vi "GUI Update Value.vi"(6 "Time":dbl, 8 "error in (no error)":errorcluster, 11 "GUI Element in":refnum<class "GUI Element.lvclass">) -> (0 "error out":errorcluster, 2 "Update":bool, 3 "GUI Element out":refnum<class "GUI Element.lvclass">, 5 "Value":variant, 7 "Control Index":i32)   [LabVIEW 2020, in "VolatusGUI.lvlib" / "GUI Element.lvclass"]
uses:
  GUI Element.lvclass
  GUI Element.lvclass/GUI Element.ctl
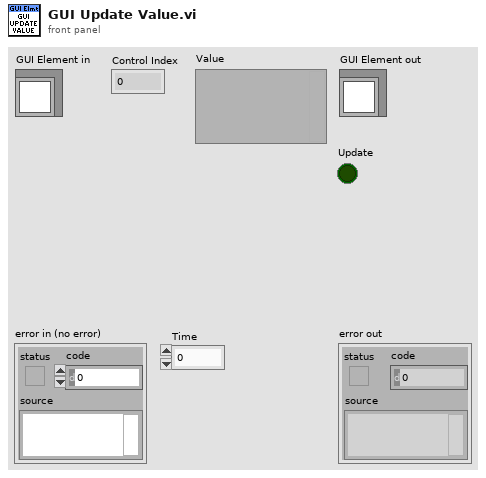
[diagram p1: front panel]
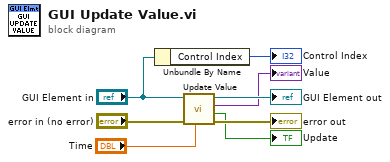
[diagram p0: block diagram]
diagram:
  n1 = Unbundle By Name("GUI Element in") -> ("Control Index"=→"Control Index":i32)
  n2 = call-dynamic "Update Value.vi"("Time"="Time", "error in (no error)"="error in (no error)", "GUI Element in"="GUI Element in") -> ("error out"=→"error out":errorcluster, "Update"=→"Update":bool, "Value"=→"Value":variant, "GUI Element out"=→"GUI Element out":refnum<class "GUI Element.lvclass">)  [unwired: 5 in]
